vi "DigitalStimToString.vi"(4 "digital stimulus":T1) -> (1 "stimulus set string":string)   [LabVIEW 2015]
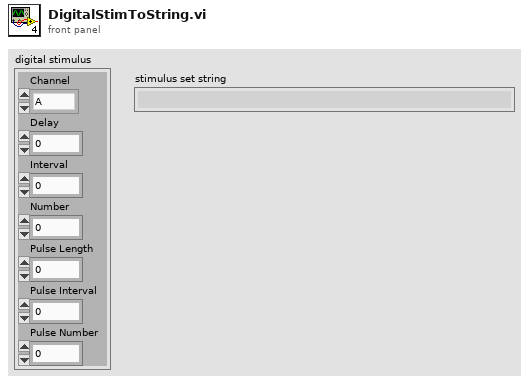
[diagram p1: front panel]
types:
  T1 = cluster{"Channel":enum16{"A", "B", "C", "D", "E", "F", "G", "H", "I", "J", "K", "L", "M", "N", "O", "P", "Q", "R", "S", "T", "U", "V", "W", "X"}, "Delay":dbl, "Interval":dbl, "Number":i32, "Pulse Length":dbl, "Pulse Interval":dbl, "Pulse Number":i32}
  T2 = enum16{"A", "B", "C", "D", "E", "F", "G", "H", "I", "J", "K", "L", "M", "N", "O", "P", "Q", "R", "S", "T", "U", "V", "W", "X"}
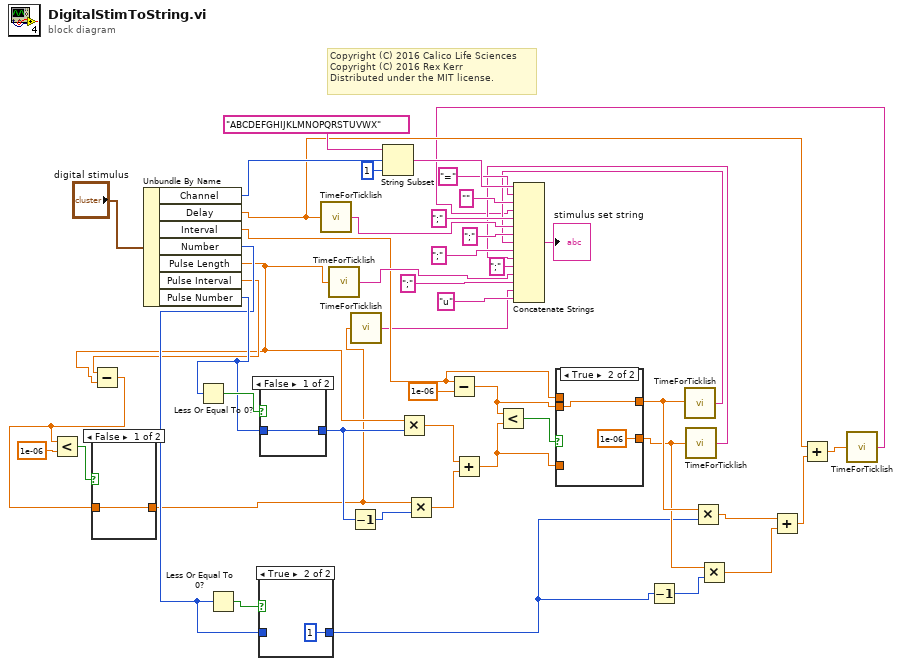
[diagram p0: block diagram]
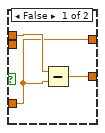
[diagram p2: hidden frame]
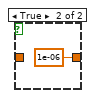
[diagram p3: hidden frame]
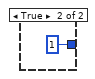
[diagram p5: hidden frame]
diagram:
  # "Copyright (C) 2016 Calico Life Sciences\nCopyright (C) 2016 Rex Kerr\nDistributed under the MIT license."
  n1 = Unbundle By Name("digital stimulus") -> ("Channel"=w46:T2, "Delay"=w4:dbl, "Interval"=w18:dbl, "Number"=w31:i32, "Pulse Length"=w22:dbl, "Pulse Interval"=w30:dbl, "Pulse Number"=w33:i32)
  n2 = Subtract(x=w30, y=w22) -> (x-y=w27:dbl)
  n3 = Less?(x=w27, y=1e-06) -> (x < y?=w28:bool)
  n4 = case shown="False" w28 {
    tunnel: w27 -> [w49 _]
    tunnel: [w49 1e-06] -> w13
    frame False {
    }
    frame True {
    }
  }
  n5 = Less Or Equal To 0?(x=w33) -> (x <= 0?=w34:bool)
  n6 = Less Or Equal To 0?(x=w31) -> (x <= 0?=w32:bool)
  n7 = case shown="True" w32 {
    tunnel: w31 -> [w51 _]
    tunnel: [w51 1 ("Number")] -> w9
    frame False {
    }
    frame True {
    }
  }
  n8 = case shown="False" w34 {
    tunnel: w33 -> [w53 _]
    tunnel: [w53 1 ("Pulse Number")] -> w26
    frame False {
    }
    frame True {
    }
  }
  n9 = call "TimeForTicklish.vi"("time"=w4) -> ("String"=w35:string)  [unwired: 4 in]
  n10 = call "TimeForTicklish.vi"("time"=w22) -> ("String"=w21:string)  [unwired: 4 in]
  n11 = Decrement(x=w26) -> (x-1=w25:i32)
  n12 = call "TimeForTicklish.vi"("time"=w13) -> ("String"=w12:string)  [unwired: 4 in]
  n13 = String Subset(string="ABCDEFGHIJKLMNOPQRSTUVWX", offset (0)=w46, length (rest)=1 ("length (rest)")) -> (substring=w37:string)
  n14 = Multiply(x=w22, y=w26) -> (x*y=w24:dbl)
  n15 = Multiply(x=w13, y=w25) -> (x*y=w23:dbl)
  n16 = Subtract(x=w18, y=1e-06) -> (x-y=w16:dbl)
  n17 = Add(x=w24, y=w23) -> (x+y=w17:dbl)
  n18 = Less?(x=w16, y=w17) -> (x < y?=w19:bool)
  n19 = case shown="True" w19 {
    tunnel: w18 -> [w56 _]
    tunnel: w17 -> [w55 _]
    tunnel: [w55 w59] -> w11
    tunnel: [w57 1e-06] -> w10
    tunnel: w16 -> [_ w59]
    frame False {
      n20 = Subtract(x=w56, y=w55) -> (x-y=w57:dbl)
    }
    frame True {
    }
  }
  n21 = Decrement(x=w9) -> (x-1=w8:i32)
  n22 = call "TimeForTicklish.vi"("time"=w11) -> ("String"=w15:string)  [unwired: 4 in]
  n23 = call "TimeForTicklish.vi"("time"=w10) -> ("String"=w14:string)  [unwired: 4 in]
  n24 = Multiply(x=w11, y=w9) -> (x*y=w7:dbl)
  n25 = Multiply(x=w10, y=w8) -> (x*y=w6:dbl)
  n26 = Add(x=w7, y=w6) -> (x+y=w5:dbl)
  n27 = Add(x=w4, y=w5) -> (x+y=w3:dbl)
  n28 = call "TimeForTicklish.vi"("time"=w3) -> ("String"=w2:string)  [unwired: 4 in]
  n29 = Concatenate Strings(w37, "=" ("string"), "" ("string"), w2, ";" ("string"), w35, ";" ("string"), w15, ";" ("string"), w14, ";" ("string"), w21, ";" ("string"), w12, "u" ("string")) -> (→"stimulus set string":string)
